vi "ComputeACPadPositions.vi"(0 "Theta Calibration":dbl format="%#_8g", 1 "X cp":dbl format="%#_8g", 2 "Y cp":dbl format="%#_8g", 4 "Sensor Path":path=path "R0Hamamatsu.txt ") -> ()   [LabVIEW 2019]
uses:
  <vilib>/Analysis/coordinate.llb/2D Cartesian Coordinate Rotation (Scalar).vi
  <vilib>/Analysis/NI_AALPro.lvlib
panel:
  out "error out":errorcluster
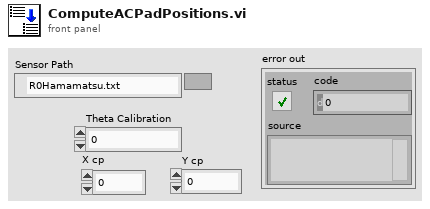
[diagram p1: front panel]
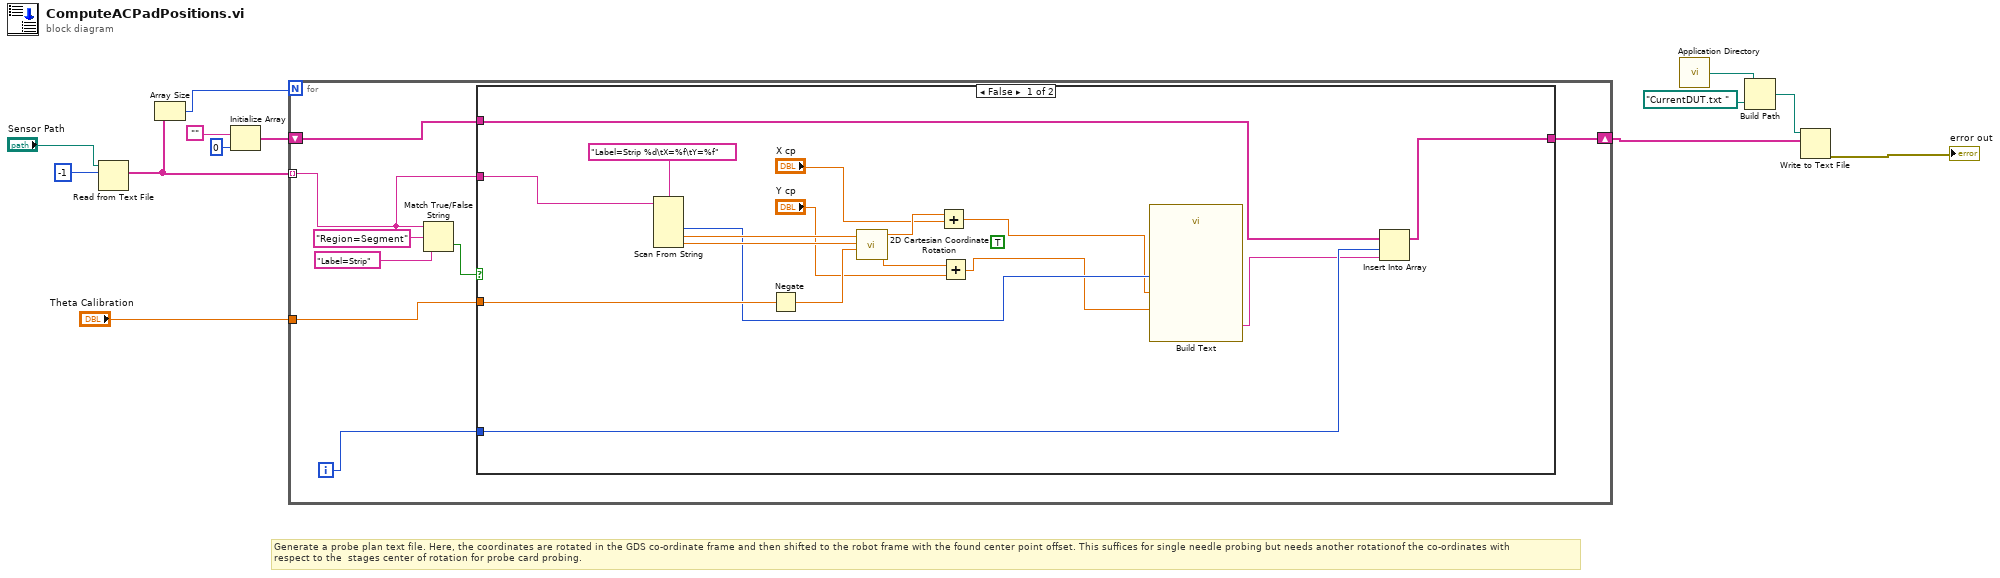
[diagram p0: block diagram]
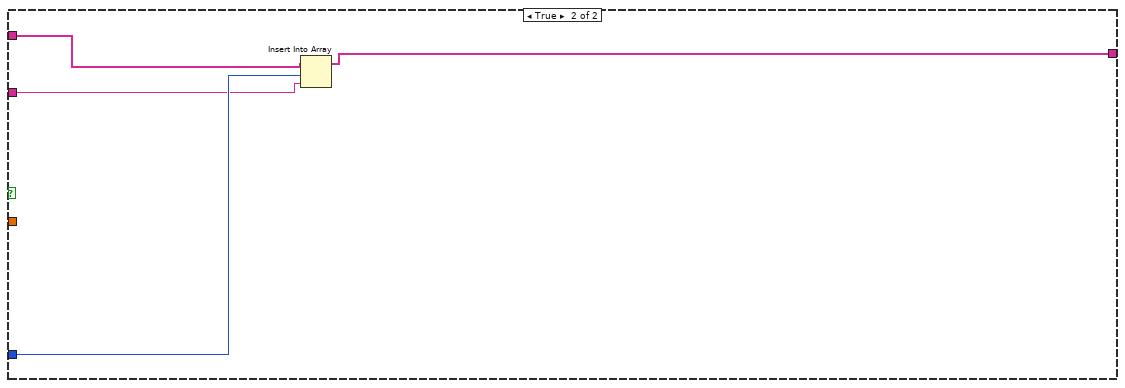
[diagram p2: hidden frame]
diagram:
  # "Generate a probe plan text file. Here, the coordinates are rotated in the GDS co-ordinate frame and then shifted to the robot frame with the found center point offset. This suffices for single needle probing but needs another rotationof the co-ordinates with\nrespect to the  stages center of rotation for probe card probing."
  n1 = Read from Text File(file (use dialog)="Sensor Path", count=-1) -> (text=w7:string[])  [unwired: 2 in, 3 out]
  n2 = Array Size(array=w7) -> (size(s)=w8:i32)
  n3 = Initialize Array("", 0 ("dimension size")) -> (w6:string[])
  n4 = for {
    N: w8 -> [_]
    tunnel: "Theta Calibration" -> [w21]
    tunnel: w7 -> [w18] mode=indexing
    shift-right: [w15] -> w3
    shift-left: w6 -> [w17]
    i -> [w16]
    n5 = Match True/False String(2:"Label=Strip" ("false string"), 3:"Region=Segment" ("true string"), 4:w18) -> (0:w19:bool)  [unwired: 1 out]
    n6 = case shown="False" w19 {
      tunnel: w21 -> [w36 _]
      tunnel: w18 -> [w34 w40]
      tunnel: w17 -> [w25 w41]
      tunnel: w16 -> [w27 w42]
      tunnel: [w24 w39] -> w15
      frame False {
        (unwired) TRUE ("Boolean")
        n7 = Scan From String(format string="Label=Strip %d\tX=%f\tY=%f", input string=w34) -> (output 1=w28:i32, output 2=w32:dbl, output 3=w31:dbl)  [unwired: 5 in, 3 out]
        n8 = Negate(x=w36) -> (-x=w35:dbl)
        n9 = call-poly <vilib>:"2D Cartesian Coordinate Rotation.vi"("theta"=w35, "y"=w31, "x"=w32) -> ("y out"=w37:dbl, "x out"=w38:dbl)  [unwired: 6 in, 1 out]
        n10 = Add(x=w38, y="X cp") -> (x+y=w23:dbl)
        n11 = Add(x=w37, y="Y cp") -> (x+y=w22:dbl)
        n12 = call "Build Text"("stripNum"=w28, "x"=w23, "y"=w22) -> ("Result"=w26:string)  [unwired: 11 in, 1 out]
        n13 = Insert Into Array(array=w25, index=w27, new element=w26) -> (w24:string[])
      }
      frame True {
        n14 = Insert Into Array(array=w41, index=w42, new element=w40) -> (w39:string[])
      }
    }
  }
  n15 = call <vilib>:"Application Directory.vi"() -> ("Application Directory"=w11:path)
  n16 = Build Path(base path=w11, name or relative path=path "CurrentDUT.txt " ("file path (dialog if empty)")) -> (appended path=w2:path)
  n17 = Write to Text File(file (use dialog)=w2, text=w3) -> (error out=→"error out":errorcluster)  [unwired: 2 in, 2 out]
